vi "Write JSON.vi"(8 "error in (no error)":errorcluster, 10 "JSON":refnum<data-value>, 11 "JSON Variable in":refnum<class "JSON Variable.lvclass">) -> (0 "error out":errorcluster, 3 "JSON Variable out":refnum<class "JSON Variable.lvclass">)   [LabVIEW 2019, in "JSON Variable.lvclass"]
uses:
  JSON Variable.lvclass
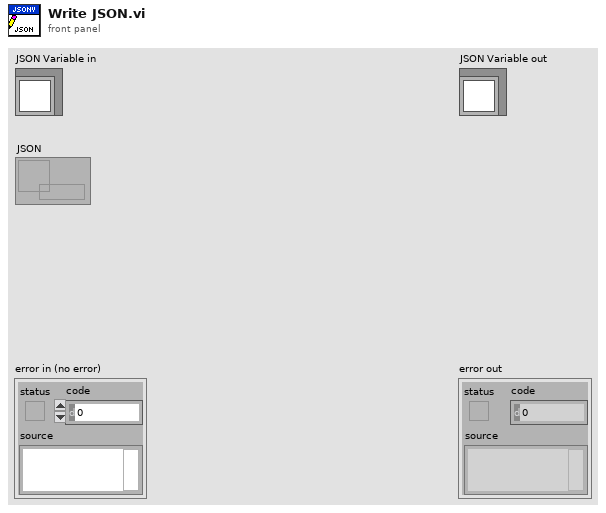
[diagram p1: front panel]
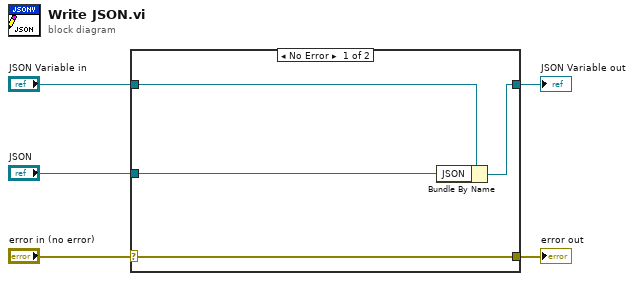
[diagram p0: block diagram]
diagram:
  n1 = case shown="No Error" "error in (no error)" {
    selector: "error in (no error)" -> [w9 w10]
    tunnel: [w9 w10] -> w4
    tunnel: [w7 w11] -> w2
    tunnel: "JSON Variable in" -> [w8 w11]
    tunnel: "JSON" -> [w6 _]
    frame No Error {
      n2 = Bundle By Name(cluster=w8, "JSON"=w6) -> (w7:refnum<class "JSON Variable.lvclass">)
    }
    frame Error {
    }
  }
  "error out" <- w4
  "JSON Variable out" <- w2
